vi "Cancelled Global.vi"() -> ()   [LabVIEW 2025]
panel:
  out "Cancelled?":bool
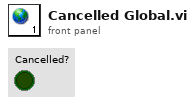
[diagram p1: front panel]
diagram:
